vi "processSubDataSubscribe.vi"(8 "error in (no error)":errorcluster, 11 "MiddlewareSALThisComponent in":refnum<class "MiddlewareSALThisComponent.lvclass">) -> (0 "error out":errorcluster, 3 "MiddlewareSALThisComponent out":refnum<class "MiddlewareSALThisComponent.lvclass">)   [LabVIEW 2016, in "MiddlewareSALThisComponent.lvclass"]
uses:
  MiddlewareSALThisComponent.lvclass
  home/andres/ct_cmpuserevents/ComponentTemplateCore/ComponentModel/ComponentModel/Middleware/Middleware.lvclass
  ComponentTemplateCore/ComponentModel/ComponentModel/Middleware/Middleware.lvclass/Middleware.ctl
  ComponentTemplateCore/ComponentModel/ComponentModel/MiddlewareProcessEvent/MiddlewareProcessEvent.lvclass/MiddlewareProcessEvent.ctl
  PubSubDataEvent/PubSubDataEvent.lvclass/PubSubDataEvent.ctl
  ComponentTemplateCore/ComponentModel/ComponentModel/Middleware/Middleware.lvclass
  ComponentTemplateCore/ComponentModel/ComponentModel/MiddlewareProcessEvent/MiddlewareProcessEvent.lvclass
  PubSubDataEvent/PubSubDataEvent.lvclass
  ts_sallv_exa/SALLV_EXA.lvlib
panel:
  out "stopIsTrue":bool
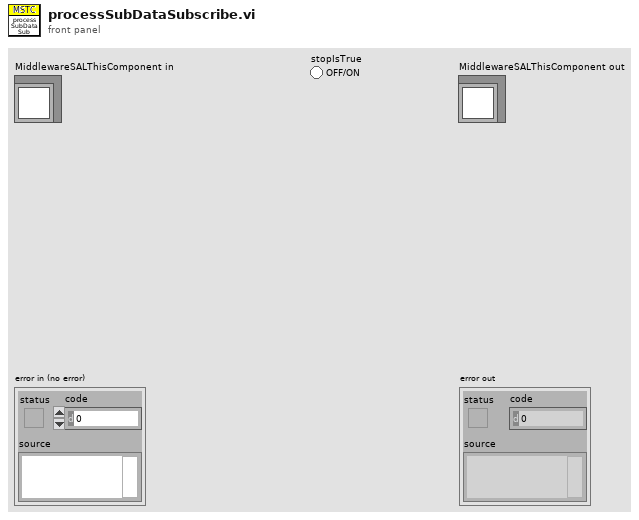
[diagram p1: front panel]
types:
  T1 = typedef "MiddlewareProcessEvents.ctl" = cluster{"disconnect":refnum<user-event>, "error":refnum<user-event>}
  T2 = cluster{"Event Registration Refnum":refnum<event-registration>, "Event Registration Refnum":refnum<event-registration>}
  T3 = typedef "EXATypedefs.lvlib/SubDataEvents.ctl" = cluster{"ClearError":refnum<user-event>, "Disable":refnum<user-event>, "Enable":refnum<user-event>, "Exit":refnum<user-event>, "GoToStandby":refnum<user-event>, "HeartbeatIn":refnum<user-event>, "Start":refnum<user-event>}
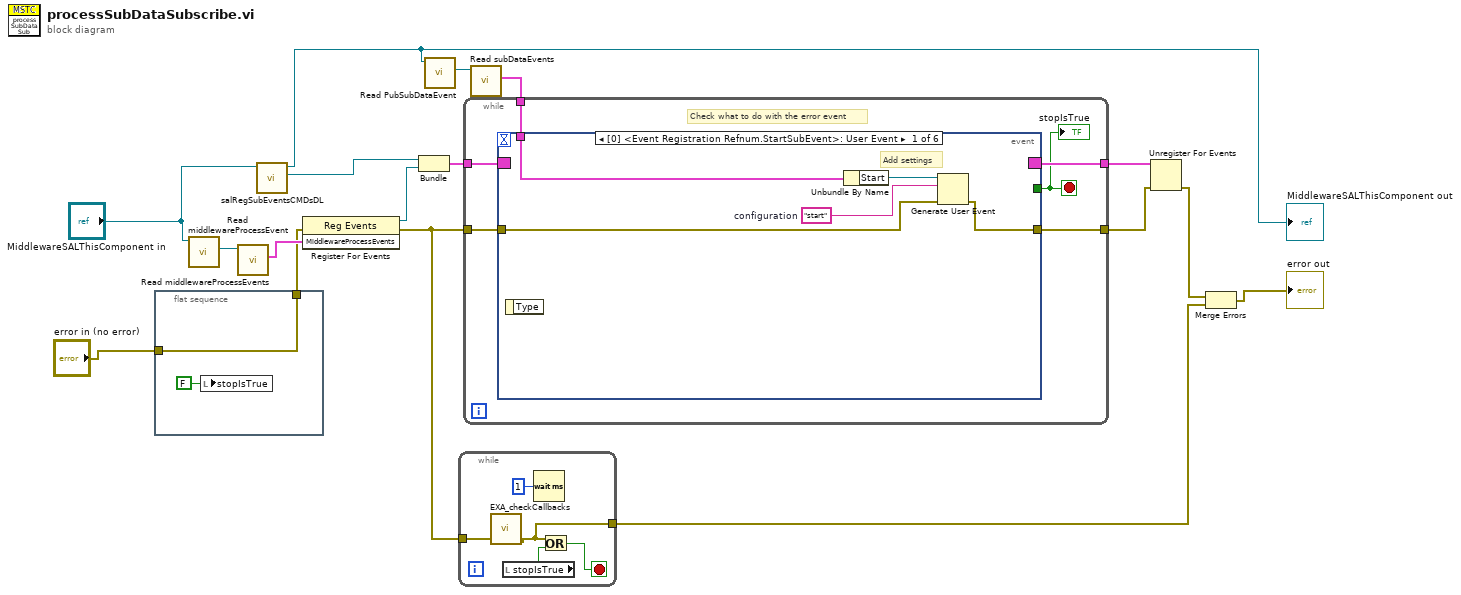
[diagram p0: block diagram]
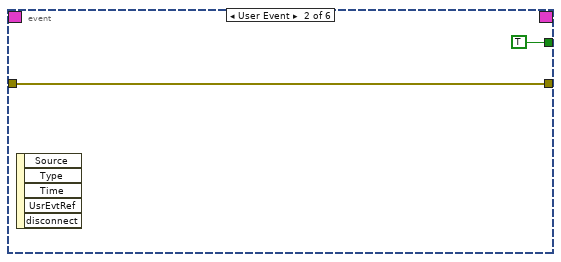
[diagram p2: hidden frame]
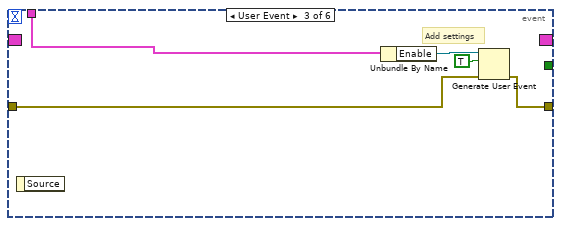
[diagram p3: hidden frame]
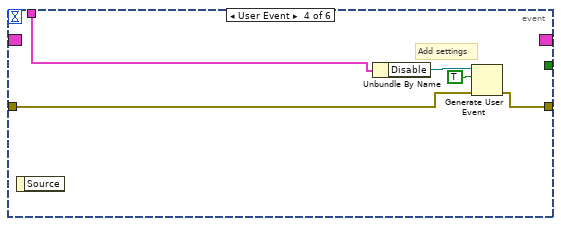
[diagram p4: hidden frame]
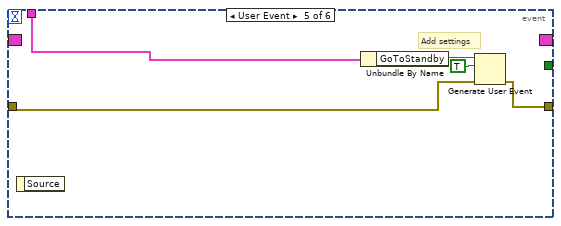
[diagram p5: hidden frame]
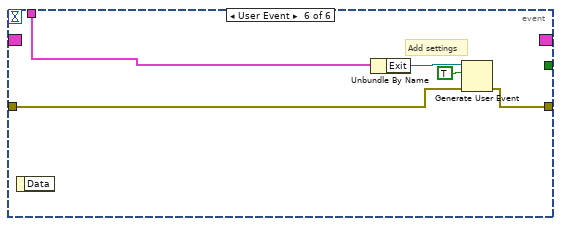
[diagram p6: hidden frame]
diagram:
  n1 = flat-sequence {
    tunnel: "error in (no error)" -> [w19]
    tunnel: [w19] -> w10
    frame #0 {
      n2 = local write "stopIsTrue"(FALSE ("stopIsTrue")) -> ()
    }
  }
  n3 = call "Read middlewareProcessEvent.vi"("Middleware in"="MiddlewareSALThisComponent in") -> ("middlewareProcessEvent"=w17:refnum<class "MiddlewareProcessEvent.lvclass">)  [unwired: 9 in, 1 out]
  n4 = call "Read middlewareProcessEvents.vi"("MiddlewareProcessEvent in"=w17) -> ("MiddlewareProcessEvents"=w16:T1)  [unwired: 9 in, 1 out]
  n5 = call "salRegSubEventsCMDsDL.vi"("MiddlewareSALThisComponent in"="MiddlewareSALThisComponent in") -> ("Event Registration Refnum"=w8:refnum<event-registration>, "MiddlewareSALThisComponent out"=w4:refnum<class "MiddlewareSALThisComponent.lvclass">)  [unwired: 8 in, 1 out]
  "MiddlewareSALThisComponent out" <- w4
  n6 = register-events(error in=w10, w16) -> (reference out=w14:refnum<event-registration>, error out=w1:errorcluster)  [unwired: 1 in]
  n7 = Bundle("Event Registration Refnum"=w8, "Event Registration Refnum"=w14) -> (w15:T2)  [unwired: 1 in]
  n8 = call-dynamic "Read PubSubDataEvent.vi"("MiddlewareSALThisComponent in"=w4) -> ("PubSubDataEvent.lvclass"=w3:refnum<class "PubSubDataEvent.lvclass">)  [unwired: 8 in, 2 out]
  n9 = while {
    tunnel: [w20] -> w5
    tunnel: w1 -> [w21]
    stop <- w22 stop-if-true
    n10 = call "EXA_checkCallbacks.vi"("error in (no error)"=w21) -> ("error out"=w20:errorcluster)  [unwired: 10 in]
    n11 = local read "stopIsTrue"() -> (w23:bool)
    n12 = Wait (ms)(milliseconds to wait=u32 1) -> ()  [unwired: 1 out]
    n13 = Or(x=w20, y=w23) -> (x .or. y?=w22:bool)
  }
  n14 = call "Read subDataEvents.vi"("PubSubDataEvent in"=w3) -> ("SubDataEvents"=w2:T3)  [unwired: 9 in, 1 out]
  n15 = while {
    tunnel: w15 -> [w30]
    tunnel: [w29] -> w13
    tunnel: w1 -> [w27]
    tunnel: [w26] -> w12
    tunnel: w2 -> [w25]
    stop <- w28 stop-if-true
    # "Check what to do with the error event"
    n16 = event shown="[0] <Event Registration Refnum.StartSubEvent>: User Event" {
      selector: w30 -> [_ _ _ _ _ _]
      dyn-events: [_ _ _ _ _ _] -> w29
      timeout: _ -> [_ _ _ _ _ _]
      tunnel: [_ TRUE ("stopIsTrue") _ _ _ _] -> w28
      tunnel: w27 -> [w33 w36 w39 w44 w49 w54]
      tunnel: [w34 w36 w40 w45 w50 w55] -> w26
      tunnel: w25 -> [w32 _ w38 w43 w48 w53]
      event User Event {
        w31 = "start"  # configuration
        # "Add settings"
        n17 = event-data() -> ()  [unwired: 1 in, 1 out]
        n18 = Unbundle By Name(w32) -> ("Start"=w35:refnum<user-event>)
        n19 = Generate User Event(user event=w35, event data cluster=w31, error in=w33) -> (error out=w34:errorcluster)  [unwired: 1 in, 1 out]
      }
      event User Event {
        n20 = event-data() -> ()  [unwired: 1 in, 5 out]
      }
      event User Event {
        # "Add settings"
        n21 = event-data() -> ()  [unwired: 1 in, 1 out]
        n22 = Unbundle By Name(w38) -> ("Enable"=w42:refnum<user-event>)
        n23 = Generate User Event(user event=w42, event data cluster=TRUE ("event data"), error in=w39) -> (error out=w40:errorcluster)  [unwired: 1 in, 1 out]
      }
      event User Event {
        # "Add settings"
        n24 = event-data() -> ()  [unwired: 1 in, 1 out]
        n25 = Unbundle By Name(w43) -> ("Disable"=w46:refnum<user-event>)
        n26 = Generate User Event(user event=w46, event data cluster=TRUE ("event data"), error in=w44) -> (error out=w45:errorcluster)  [unwired: 1 in, 1 out]
      }
      event User Event {
        # "Add settings"
        n27 = event-data() -> ()  [unwired: 1 in, 1 out]
        n28 = Unbundle By Name(w48) -> ("GoToStandby"=w51:refnum<user-event>)
        n29 = Generate User Event(user event=w51, event data cluster=TRUE ("event data"), error in=w49) -> (error out=w50:errorcluster)  [unwired: 1 in, 1 out]
      }
      event User Event {
        # "Add settings"
        n30 = event-data() -> ()  [unwired: 1 in, 1 out]
        n31 = Unbundle By Name(w53) -> ("Exit"=w57:refnum<user-event>)
        n32 = Generate User Event(user event=w57, event data cluster=TRUE ("event data"), error in=w54) -> (error out=w55:errorcluster)  [unwired: 1 in, 1 out]
      }
    }
    "stopIsTrue" <- w28
  }
  n33 = Unregister For Events(event registration refnum=w13, error in=w12) -> (error out=w7:errorcluster)
  n34 = Merge Errors(w7, w5) -> (→"error out":errorcluster)
